vi "Help Scaling.vi"() -> ()   [LabVIEW 2015]
panel:
  in  "stop":bool
  # "Help"
  # "Sensor Calibration Method"
  # "1.   Select the Instrument from the Select For Calibration, to which you want to calibrate.\n\n2. Write the Value of Voltage in First Cell of Input Values. Old Calibrated Value in the \n     coressponding cell will automatically be shown, Now write the Value in the same number\n     of cell in New Calibrated Value you want to see for the Voltage You write in Input Values.\n\n3. Now press the Next Button and do the same for next cell of Input values, Old calibrated \n    Values and New Calibrated Value.\n\n4. If done with all 5 cells then press Calibrate and Save to take effect of these Values.\n\n5. Now to calibrate any other instrument select that instrument from Select for Calibration \n    and repeat step 1 to 4.\n\n6. If calibration is done then press Quit."
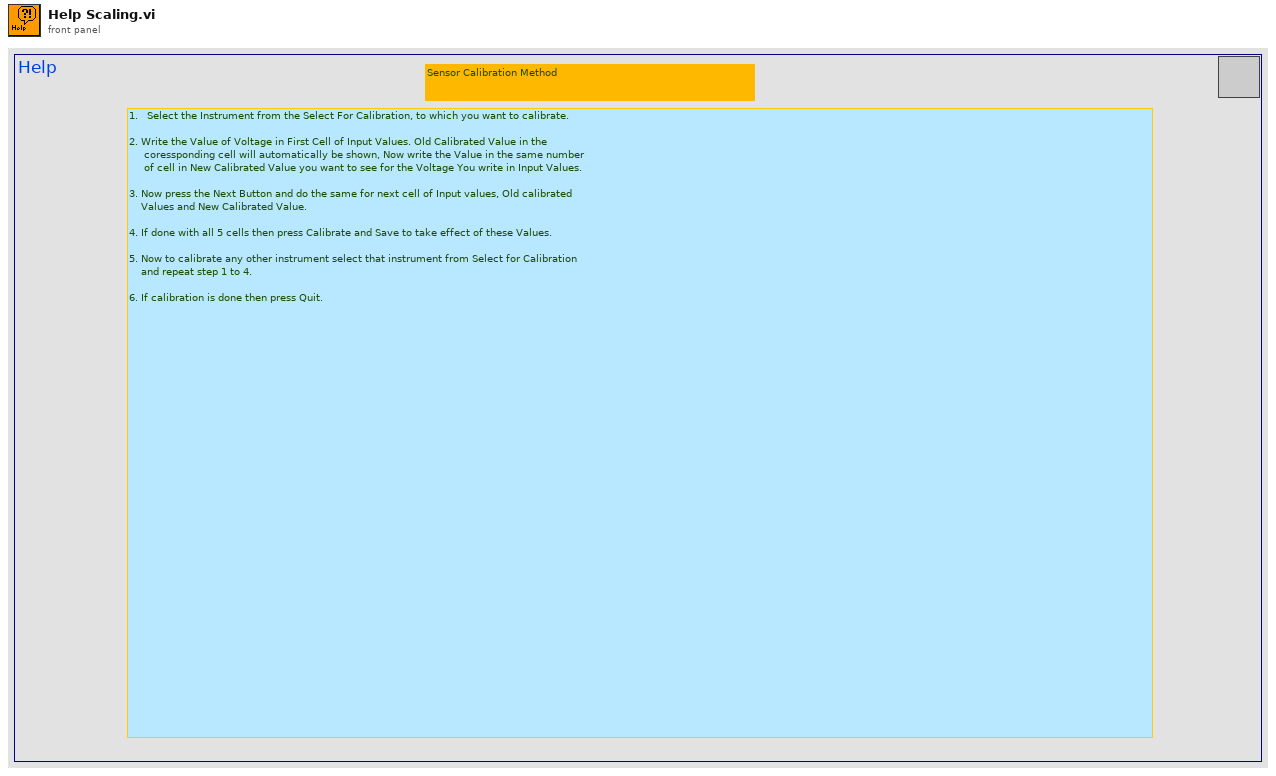
[diagram p1: front panel]
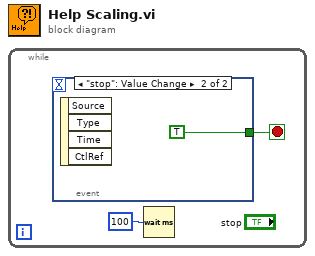
[diagram p0: block diagram]
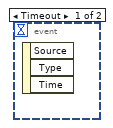
[diagram p2: hidden frame]
diagram:
  n1 = while {
    stop <- w2 stop-if-true
    n2 = event shown="[1] \"stop\": Value Change" {
      selector: _ -> [_ _]
      dyn-events: _ -> [_ _]
      timeout: _ -> [_ _]
      tunnel: [_ TRUE] -> w2
      event Timeout {
        n3 = event-data() -> ()  [unwired: 1 in, 3 out]
      }
      event "stop": Value Change {
        n4 = event-data() -> ()  [unwired: 1 in, 4 out]
      }
    }
    n5 = Wait (ms)(milliseconds to wait=u32 100) -> ()  [unwired: 1 out]
  }
